vi "NF WF1973_74 TST.vi"(8 "error in (no error)":errorcluster caption="Error IN", 11 "VISAsession":refnum<visa-resource-name>) -> (0 "error out":errorcluster caption="Error OUT", 2 "Query TST":i32, 3 "CopyVISAsession":refnum<visa-resource-name>)   [LabVIEW 2010]
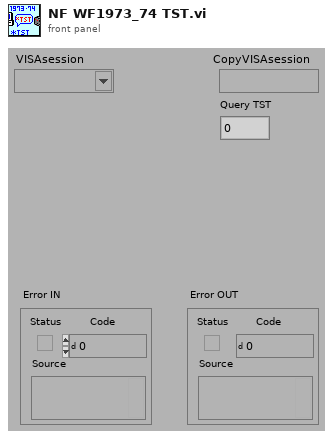
[diagram p1: front panel]
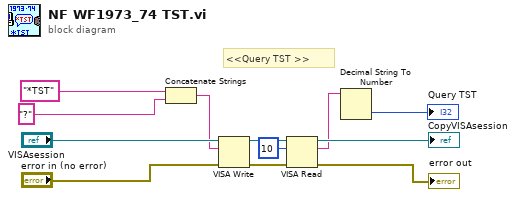
[diagram p0: block diagram]
diagram:
  # "<<Query TST >>"
  n1 = Concatenate Strings("*TST" ("文字列"), "?" ("形式文字列")) -> (w2:string)
  n2 = VISA Write(VISA resource name="VISAsession", write buffer=w2, error in (no error)="error in (no error)") -> (VISA resource name out=w5:refnum<visa-resource-name>, error out=w6:errorcluster)  [unwired: 1 out]
  n3 = VISA Read(VISA resource name=w5, byte count=u32 10 ("バイトカウント（0）"), error in (no error)=w6) -> (VISA resource name out=→"CopyVISAsession":refnum<visa-resource-name>, read buffer=w1:string, error out=→"error out":errorcluster)  [unwired: 1 out]
  n4 = Decimal String To Number(string=w1) -> (number=→"Query TST":i32)  [unwired: 2 in, 1 out]
